vi "test.ExitInfiniteLoop.vi"(8 "error in":errorcluster) -> (0 "error out":errorcluster)   [LabVIEW 2014]
uses:
  Private/Class/meth.Constructor.vi
  Private/Class/meth.Destructor.vi
  GLue.lvlib
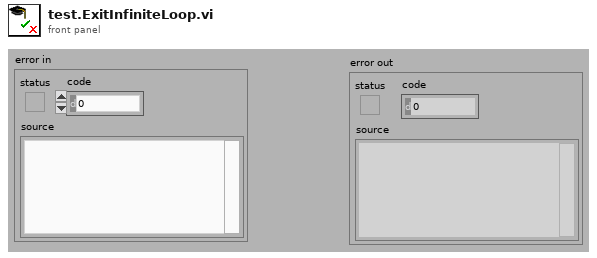
[diagram p1: front panel]
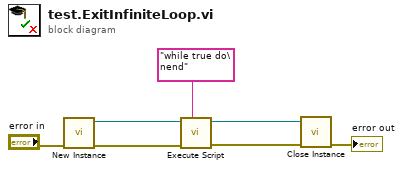
[diagram p0: block diagram]
diagram:
  n1 = call "New Instance.vi"("error in"="error in") -> ("error out"=w5:errorcluster, "GLue out"=w4:refnum<class "class.GLue.lvclass">)  [unwired: 9 in]
  n2 = call "Execute Script.vi"("Script"="while true do\nend", "error in"=w5, "GLue in"=w4) -> ("error out"=w2:errorcluster, "GLue out"=w3:refnum<class "class.GLue.lvclass">)  [unwired: 6 in, 1 out]
  n3 = call "Close Instance.vi"("error in"=w2, "GLue in"=w3) -> ("error out"=→"error out":errorcluster)  [unwired: 9 in]
